vi "AddClass.vi"(9 "Count":i32, 11 "Math.lvclass":refnum<class "Math.lvclass">) -> (3 "Math.lvclass out":refnum<class "Math.lvclass">)   [LabVIEW 2016, in "Math.lvclass"]
uses:
  Math.lvclass
  Math.lvclass/Math.ctl
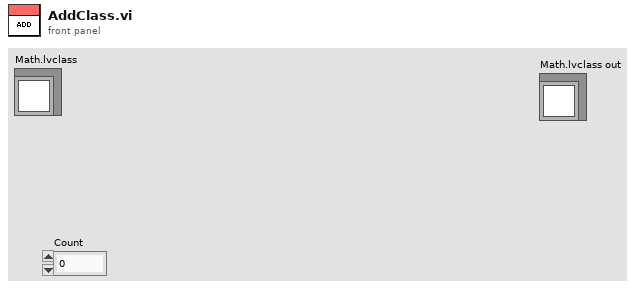
[diagram p1: front panel]
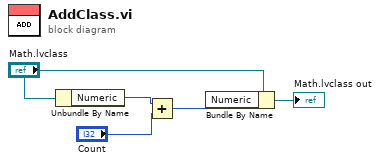
[diagram p0: block diagram]
diagram:
  n1 = Unbundle By Name("Math.lvclass") -> ("Numeric"=w5:i32)
  n2 = Add(x=w5, y="Count") -> (x+y=w2:i32)
  n3 = Bundle By Name(cluster="Math.lvclass", "Numeric"=w2) -> (→"Math.lvclass out":refnum<class "Math.lvclass">)
